vi "Config Correct Cable.vi"(0 "VISA resource name":refnum<visa-resource-name>, 1 "Length (1.00 m)":dbl=1.0 min=0.0 max=1000.0 step=0.01 format="%.2f", 2 "Resistance (40.0 milliohm/m)":dbl=40.0 min=0.0 max=9999.0 step=0.1 format="%.1f", 3 "Inductance (1.10 microhenry/m)":dbl=1.1 min=0.0 max=100.0 step=0.01 format="%.2f", 4 "Capacitance (100.0 pF/m)":dbl=100.0 min=0.0 max=1000.0 step=0.1 format="%.1f", 5 "error in":errorcluster) -> (14 "VISA resource name out":refnum<visa-resource-name>, 19 "error out":errorcluster)   [LabVIEW 2019, in "Andeen-Hagerling 2700(400 firmware).lvlib"]
doc: "Compensates for the characteristics of longer cables or cables used to connect the bridge to larger capacitances. This command is only enabled on Option-E bridges when Cor_Type is set to CABLE."
uses:
  Andeen-Hagerling 2700(400 firmware).lvlib
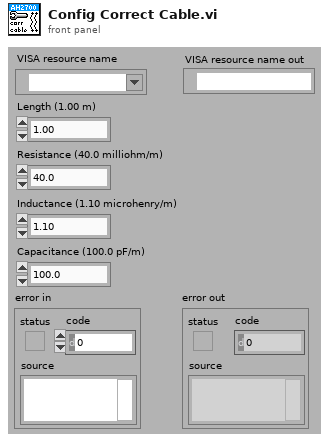
[diagram p1: front panel]
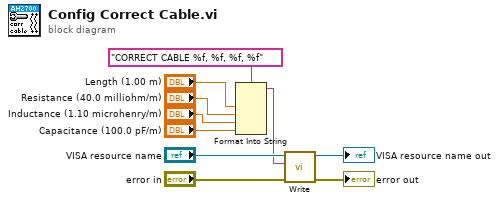
[diagram p0: block diagram]
diagram:
  n1 = Format Into String(format string="CORRECT CABLE %f, %f, %f, %f", "Length (1.00 m)", "Resistance (40.0 milliohm/m)", "Inductance (1.10 microhenry/m)", "Capacitance (100.0 pF/m)") -> (resulting string=w2:string)  [unwired: 2 in, 1 out]
  n2 = call "Write.vi"("error in"="error in", "command"=w2, "VISA resource name"="VISA resource name") -> ("error out"=→"error out":errorcluster, "VISA resource name out"=→"VISA resource name out":refnum<visa-resource-name>)  [unwired: 7 in]
